vi "Send Single Message To Specific Target.vi"(8 "error in (no error)":errorcluster, 9 "Mail Strategy In":refnum<class "Mail Strategy.lvclass">, 10 "Message In":refnum<class "Message.lvclass">, 11 "Messenger in":refnum<class "Simple Tree Queue Messenger.lvclass">) -> (0 "error out":errorcluster, 3 "Messenger out":refnum<class "Simple Tree Queue Messenger.lvclass">)   [LabVIEW 2019, in "Simple Tree Queue Messenger.lvclass"]
uses:
  Simple Tree Queue Messenger.lvclass
  C:/Users/iio/Desktop/MultiSPIM/General Library/Ancestor Class/Messenger/Messenger Composite/Messenger Composite.lvclass
  Ancestor Class/Messenger/Mail Strategy/Mail Strategy.lvclass
  Ancestor Class/Message/Message.lvclass
  Simple Tree Queue Mailman/Simple Tree Queue Mailman.lvclass
  C:/Users/iio/Desktop/MultiSPIM/General Library/Ancestor Class/Messenger/Mail Strategy/Mail Strategy.lvclass
  Ancestor Class/Messenger/Messenger Composite/Messenger Composite.lvclass/Messenger Composite.ctl
  Simple Tree Queue Mailman/Simple Tree Queue Mailman.lvclass/Simple Tree Queue Mailman.ctl
  Simple Tree Queue Messenger.lvclass/Simple Tree Queue Messenger.ctl
  Simple Tree Queue Mailman/Public Data/Write Address Recursive Access.vi
  Ancestor Class/Messenger/Messenger Composite/Public Data/Read Nodes.vi
  Ancestor Class/Messenger/Messenger/Messenger.lvclass
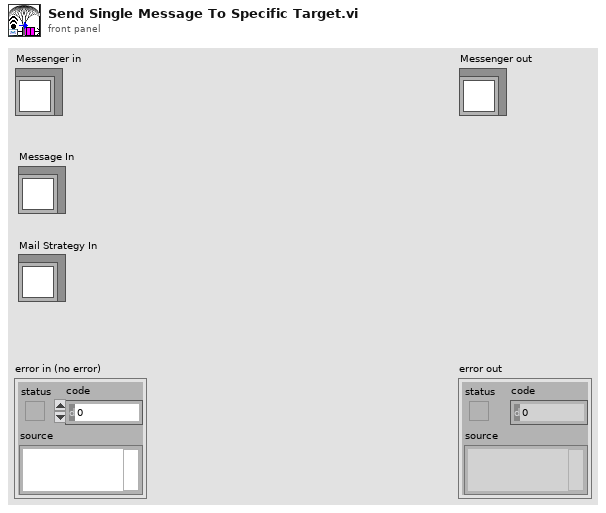
[diagram p1: front panel]
types:
  T1 = typedef "Message Queue.ctl" = refnum<queue>
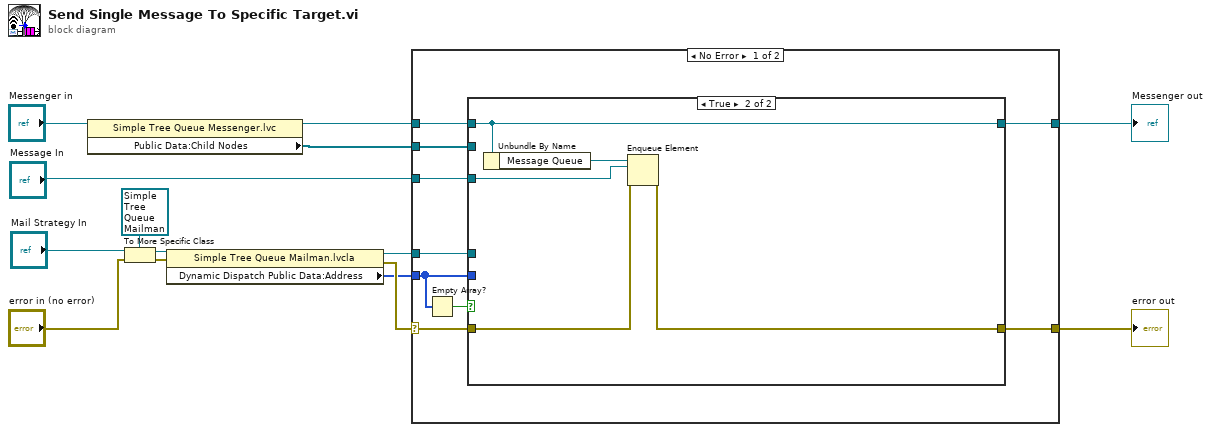
[diagram p0: block diagram]
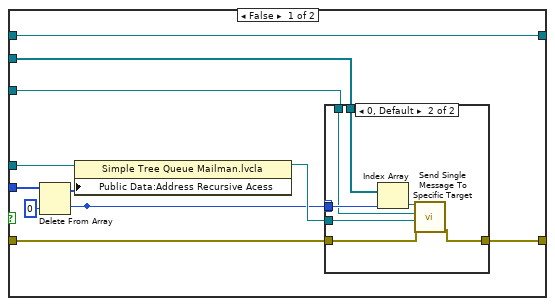
[diagram p2: hidden frame]
diagram:
  n1 = property class="Simple Tree Queue Messenger.lvc"(reference="Messenger in") -> (reference out=w5:refnum<class "Simple Tree Queue Messenger.lvclass">, "Public Data:Child Nodes"=w4:refnum<class "Messenger.lvclass">[])  [unwired: 1 in, 1 out]
  n2 = To More Specific Class(target class=refnum<class "Simple Tree Queue Mailman.lvclass"> refnum ("Array Location Mailman.lvclass"), reference="Mail Strategy In", error in="error in (no error)") -> (specific class reference=w9:refnum<class "Simple Tree Queue Mailman.lvclass">, error out=w10:errorcluster)
  n3 = property class="Simple Tree Queue Mailman.lvcla"(reference=w9, error in=w10) -> (reference out=w3:refnum<class "Simple Tree Queue Mailman.lvclass">, error out=w8:errorcluster, "Dynamic Dispatch Public Data:Address"=w1:i32[])
  n4 = case shown="No Error" w8 {
    selector: w8 -> [w18 w48]
    tunnel: w5 -> [w22 w49]
    tunnel: [w20 w49] -> w14
    tunnel: [w17 w48] -> w13
    tunnel: w1 -> [w19 _]
    tunnel: "Message In" -> [w21 _]
    tunnel: w4 -> [w16 _]
    tunnel: w3 -> [w15 _]
    frame No Error {
      n5 = Empty Array?(array=w19) -> (empty?=w23:bool)
      n6 = case shown="True" w23 {
        tunnel: w22 -> [w34 w43]
        tunnel: w21 -> [w24 w46]
        tunnel: [w34 w43] -> w20
        tunnel: w19 -> [w33 _]
        tunnel: w18 -> [w27 w45]
        tunnel: [w26 w44] -> w17
        tunnel: w16 -> [w31 _]
        tunnel: w15 -> [w30 _]
        frame False {
          n7 = Delete From Array(array=w33, index=0) -> (deleted portion=w25:i32, array with subset deleted=w29:i32[])  [unwired: 1 in]
          n8 = property class="Simple Tree Queue Mailman.lvcla"(reference=w30, "Public Data:Address Recursive Acess"=w29) -> (reference out=w28:refnum<class "Simple Tree Queue Mailman.lvclass">)  [unwired: 1 in, 1 out]
          n9 = case shown="0, Default" w25 {
            tunnel: w25 -> [_ w42]
            tunnel: w31 -> [_ w41]
            tunnel: w28 -> [_ w39]
            tunnel: w27 -> [w35 w38]
            tunnel: [w35 w37] -> w26
            tunnel: w24 -> [_ w36]
            frame -2147483648..-1 {
            }
            frame 0, Default {
              n10 = Index Array(array=w41, index=w42) -> (element=w40:refnum<class "Messenger.lvclass">)
              n11 = call-dynamic "Send Single Message To Specific Target.vi"("error in (no error)"=w38, "Mail Strategy In"=w39, "Message In"=w36, "Messenger in"=w40) -> ("error out"=w37:errorcluster)  [unwired: 6 in, 1 out]
            }
          }
        }
        frame True {
          n12 = Unbundle By Name(w43) -> ("Message Queue"=w47:T1)
          n13 = Enqueue Element(queue=w47, element=w46, error in (no error)=w45) -> (error out=w44:errorcluster)  [unwired: 1 in, 2 out]
        }
      }
    }
    frame Error {
    }
  }
  "error out" <- w13
  "Messenger out" <- w14
